vi "GL_heaterInput.vi"() -> ()   [LabVIEW 2021]
panel:
  in  "Array 2":bool[](array[boolean])
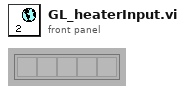
[diagram p1: front panel]
diagram:
